vi "SUB_SEARCH_REPLACE_STR.vi"(3 "replace string (\"\")":string, 4 "search string":string, 5 "input string":string) -> (2 "result string":string)   [LabVIEW 2011]
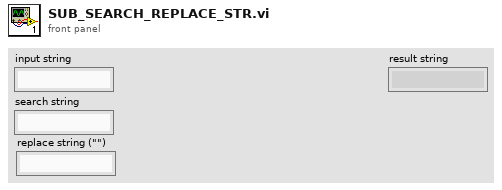
[diagram p1: front panel]
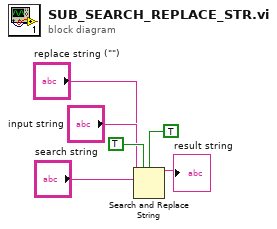
[diagram p0: block diagram]
diagram:
  n1 = Search and Replace String(replace all?=TRUE ("replace all? (F)"), case sensitive?=TRUE ("ignore case? (F)"), input string="input string", search string="search string", replace string="replace string (\"\")") -> (result string=→"result string":string)  [unwired: 3 in, 3 out]
